vi "updateShoot.vi"(10 "Shooting Time":u32) -> (3 "Boolean":bool)   [LabVIEW 2014]
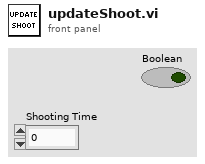
[diagram p1: front panel]
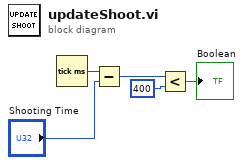
[diagram p0: block diagram]
diagram:
  n1 = Tick Count (ms)() -> (millisecond timer value=w4:u32)
  n2 = Subtract(x=w4, y="Shooting Time") -> (x-y=w2:u32)
  n3 = Less?(x=w2, y=u32 400) -> (x < y?=→"Boolean":bool)
